vi "FT_Get_Device_Description_By_Index.vi"(8 "error in":errorcluster, 11 "Device Index":u32) -> (0 "error out":errorcluster, 3 "Device Description":string)   [LabVIEW 2016]
uses:
  FTD2XX.dll
panel:
  # "Get device description by index.\n\nNOTE: device index is 0 based"
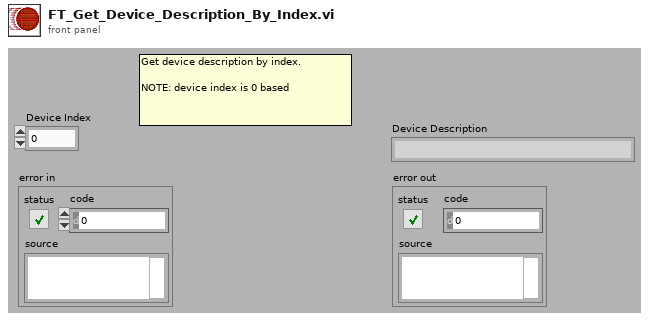
[diagram p1: front panel]
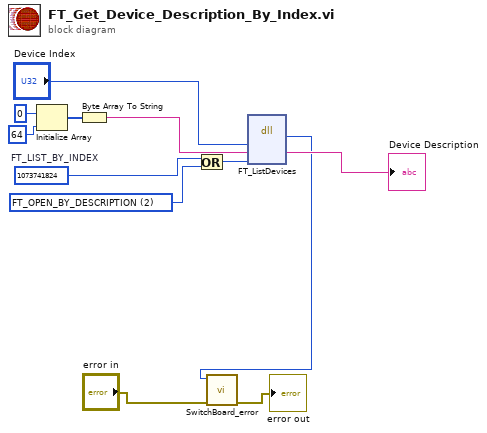
[diagram p0: block diagram]
diagram:
  w10 = u32 2 items=["FT_OPEN_BY_SERIAL_NUMBER"=1, "FT_OPEN_BY_DESCRIPTION"=2, "FT_OPEN_BY_LOCATION"=4] ("Flags")
  w9 = u32 1073741824  # FT_LIST_BY_INDEX
  n1 = Initialize Array(u8 0, 64 ("dimension size")) -> (w6:u8[])
  n2 = Byte Array To String(unsigned byte array=w6) -> (string=w5:string)
  n3 = Or(x=w9, y=w10) -> (x .or. y?=w8:u32)
  n4 = dll-call lib="FTD2XX.dll" fn="FT_ListDevices"("DeviceIndex"="Device Index", "DeviceDescription"=w5, "Flags"=w8) -> ("FT_Status"=w1:u32, "DeviceDescription"=→"Device Description":string)  [unwired: 5 in, 2 out]
  n5 = call <instrlib>:"SwitchBoard_error.vi"("error constant"="error in", "Code"=w1) -> ("error IO"=→"error out":errorcluster)  [unwired: 9 in]
